vi "Tool_Unicode Update String Array (2D).vi"(5 "Interpret as Unicode (T)":bool=TRUE, 6 "error in (no error)":errorcluster, 7 "Caption":string, 8 "Value":string[][](array[string]), 9 "String Array (2D) Ref":refnum<vi>) -> (0 "error out":errorcluster, 3 "String Array (2D) Ref":refnum<vi>)   [LabVIEW 2009]
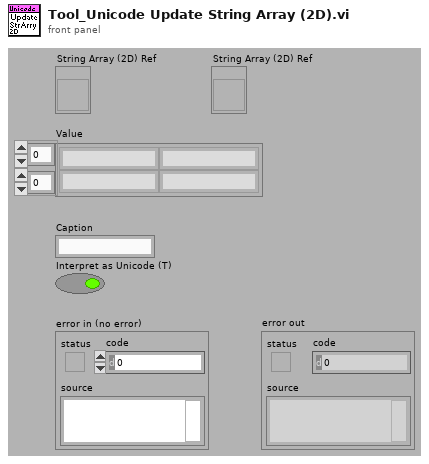
[diagram p1: front panel]
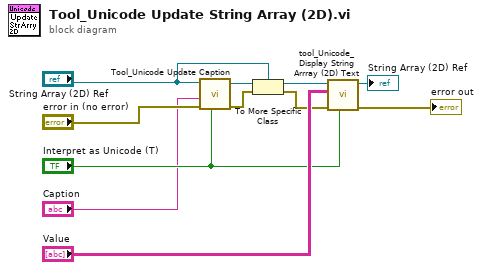
[diagram p0: block diagram]
diagram:
  n1 = call "Tool_Unicode Update Caption.vi"("Interpret as Unicode (T)"="Interpret as Unicode (T)", "error in (no error)"="error in (no error)", "Caption"="Caption", "Control Reference"="String Array (2D) Ref") -> ("error out"=w7:errorcluster, "Control Reference"=w6:refnum<vi>)  [unwired: 4 in]
  n2 = To More Specific Class(target class="String Array (2D) Ref", reference=w6, error in=w7) -> (specific class reference=w4:refnum<vi>, error out=w5:errorcluster)
  n3 = call "tool_Unicode_Display String Arrray (2D) Text.vi"("Interpret as Unicode (T)"="Interpret as Unicode (T)", "error in"=w5, "Value"="Value", "String Array (2D) Ref"=w4) -> ("error out"=→"error out":errorcluster, "String Array (2D) Ref"=→"String Array (2D) Ref":refnum<vi>)  [unwired: 4 in]
